vi "Self-Cal.vi"(8 "error in (no error)":errorcluster, 11 "DAQmx Base in":refnum<class "NI DAQmx Base.lvclass">) -> (0 "error out":errorcluster, 2 "Result":variant, 3 "DAQmx Base out":refnum<class "NI DAQmx Base.lvclass">)   [LabVIEW 2020, in "NI DAQmx.lvlib" / "NI DAQmx Base.lvclass"]
uses:
  NI DAQmx Base.lvclass
  NI DAQmx Base.lvclass/NI DAQmx Base.ctl
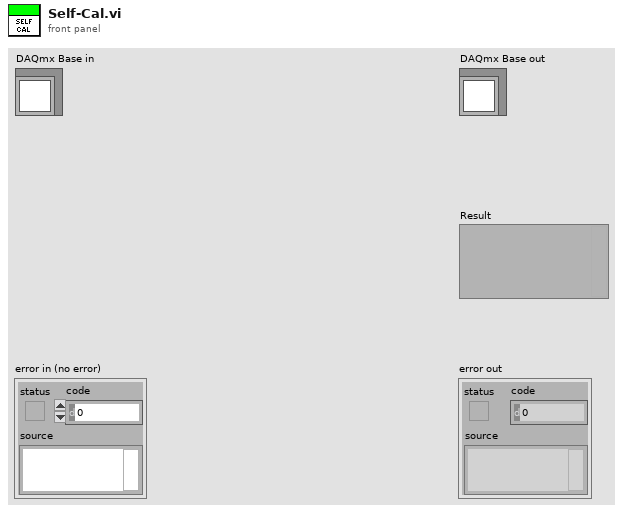
[diagram p1: front panel]
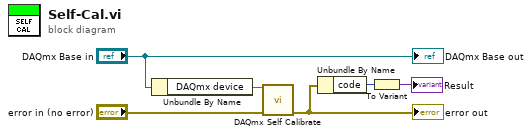
[diagram p0: block diagram]
diagram:
  n1 = Unbundle By Name("DAQmx Base in") -> ("DAQmx device"=w6:tag)
  n2 = call <vilib>:"DAQmx Self Calibrate.vi"("device in"=w6, "error in"="error in (no error)") -> ("error out"=w2:errorcluster)  [unwired: 13 in]
  "error out" <- w2
  n3 = Unbundle By Name(w2) -> ("code"=w5:i32)
  n4 = To Variant(anything=w5) -> (Variant=→"Result":variant)
  "DAQmx Base out" <- "DAQmx Base in"
